vi "SV Compute Statistical Level from Buffered Array.vi"(0 "data":dbl[](array[numeric]), 5 "N (50 %)":dbl=50.0 min=0.0 max=100.0 step=0.5) -> (4 "sorted data":dbl[](array[numeric]), 6 "L_N":dbl=nan min=0.0 max=100.0 step=0.5 format="%_4g")   [LabVIEW 2017]
doc: "Use this VI to return <B>L_N</B> levels where L_N is the level which N % of the values exceed. For example, L50 represents the median, where 50 % of the values are greater than L_N and 50 % are lower. L90 is commonly used as a noise baseline, as 90 % of the values exceed L_N. L10 is commonly used as a measure of peak levels because it corresponds to the highest 10 % of levels."
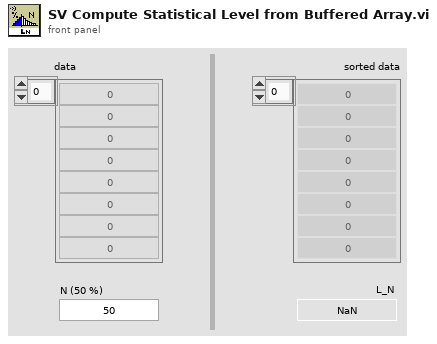
[diagram p1: front panel]
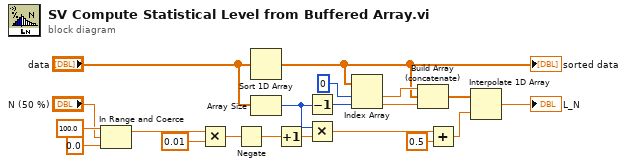
[diagram p0: block diagram]
diagram:
  n1 = In Range and Coerce(upper limit=100.0, x="N (50 %)", lower limit=0.0) -> (coerced(x)=w13:dbl)  [unwired: 1 out]
  n2 = Multiply(x=w13, y=0.01 ("x")) -> (x*y=w19:dbl)
  n3 = Negate(x=w19) -> (-x=w18:dbl)
  n4 = Sort 1D Array(array="data") -> (sorted array=w6:dbl[])
  "sorted data" <- w6
  n5 = Array Size(array="data") -> (size(s)=w8:i32)
  n6 = Increment(x=w18) -> (x+1=w17:dbl)
  n7 = Decrement(x=w8) -> (x-1=w9:i32)
  n8 = Multiply(x=w8, y=w17) -> (x*y=w12:dbl)
  n9 = Index Array(array=w6, index #1=0 ("index"), index #2=w9) -> (element #1=w7:dbl, element #2=w5:dbl)
  n10 = Build Array (concatenate)(w7, w6, w5) -> (w4:dbl[])
  n11 = Add(x=w12, y=0.5) -> (x+y=w3:dbl)
  n12 = Interpolate 1D Array(1:w3, 2:w4) -> (0:→"L_N":dbl)
